vi "Resetable filter.vi"() -> ()   [LabVIEW 2009]
uses:
  <vilib>/ptbypt/NI_PtbyPt.lvlib
panel:
  in  "Numeric 2":i32=100 min=10 step=20
  out "Gauge":dbl(knob) scale=0.0..1.0
  in  "stop":bool
  out "Numeric":dbl=100.0 format="%#_10f"
  out "Boolean":bool
  in  "OK Button":bool
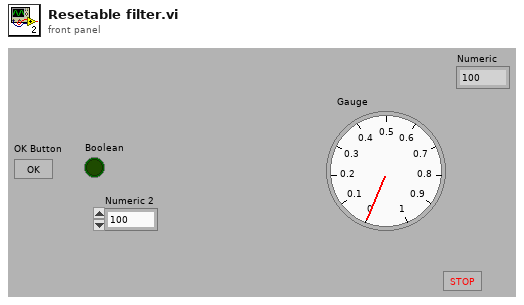
[diagram p1: front panel]
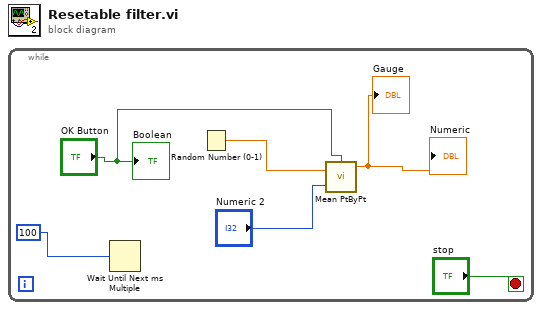
[diagram p0: block diagram]
diagram:
  n1 = while {
    stop <- "stop" stop-if-true
    n2 = Wait Until Next ms Multiple(millisecond multiple=100) -> ()  [unwired: 1 out]
    n3 = Random Number (0-1)() -> (number: 0 to 1=w5:dbl)
    n4 = call <vilib>:"Mean PtByPt.vi"("x"=w5, "sample length"="Numeric 2", "initialize"="OK Button") -> ("mean"=→"Numeric" →"Gauge":dbl)  [unwired: 2 out]
    "Boolean" <- "OK Button"
  }
